vi "Harry_kane_CDR.vi"() -> ()   [LabVIEW 2013]
uses:
  <vilib>/vision/Image Controls.llb/IMAQ Image.ctl
  <vilib>/vision/driver/NI_Vision_Acquisition_Software.lvlib
panel:
  in  "Boolean":bool
  in  "stop":bool
  in  "Player area overlay":T1
  out "Puck and player location":T1(plugin-control)
  out "Player Array From Reference":dbl[][](array[numeric])
  out "Puck Array From Reference":dbl[][](array[numeric])
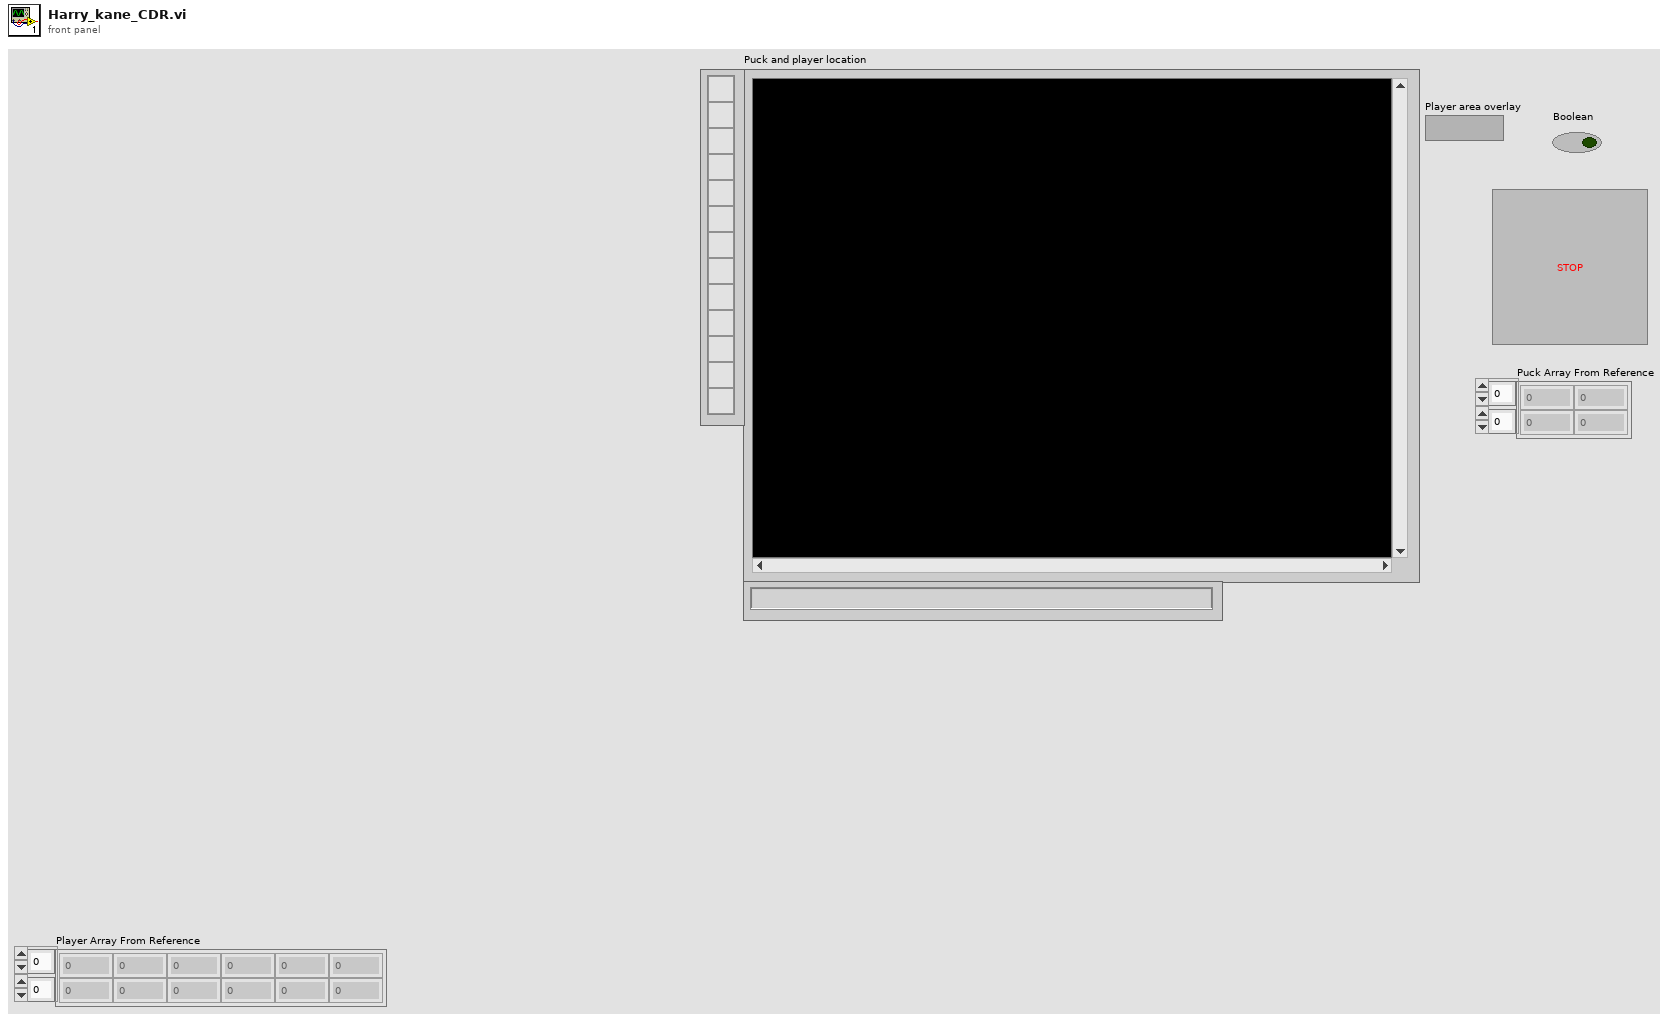
[diagram p1: front panel]
types:
  T1 = typedef "IMAQ Image.ctl" = refnum<image>
  T2 = typedef "Image Type" = u32
  T3 = typedef "IMAQdx.ctl" = refnum<k21>
  T4 = cluster{"Point1 (Pixels)":cluster{"X":sgl, "Y":sgl}, "Point2 (Pixels)":cluster{"X":sgl, "Y":sgl}, "Point1 (Real-World)":cluster{"X":sgl, "Y":sgl}, "Point2 (Real-World)":cluster{"X":sgl, "Y":sgl}, "Angle (Pixel)":dbl, "Angle (Real-World)":dbl, "Score":dbl, "Straightness":dbl, "Average SNR (db)":dbl, "Calibration Valid":bool}
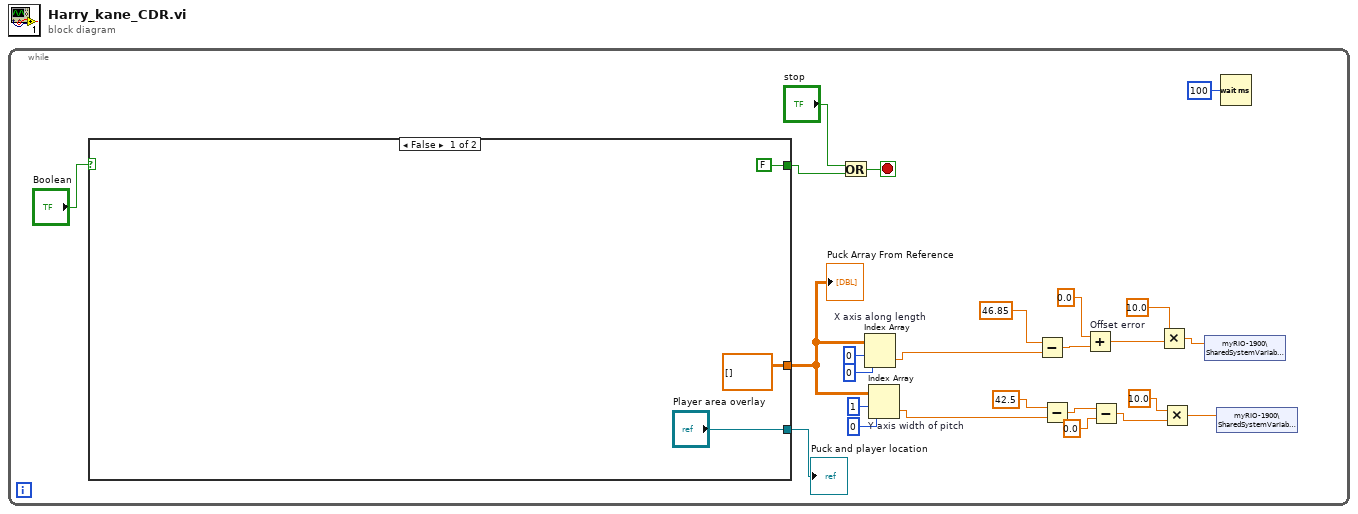
[diagram p0: block diagram]
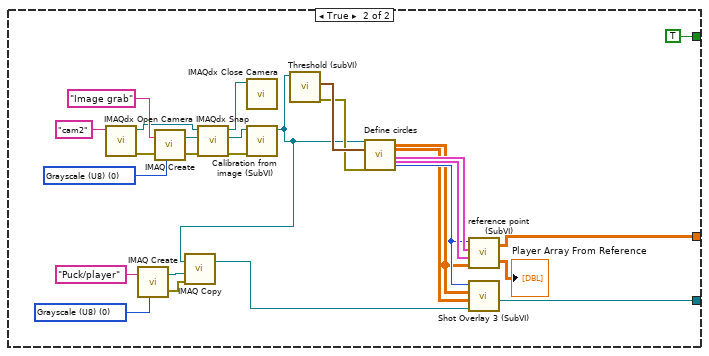
[diagram p2: hidden frame]
diagram:
  n1 = while {
    stop <- w15 stop-if-true
    n2 = case shown="False" "Boolean" {
      tunnel: ["Player area overlay" w37] -> w25
      tunnel: [dbl[][] [] ("Puck X, Y co-ordinates") w36] -> w22
      tunnel: [FALSE ("x") TRUE ("x")] -> w16
      frame False {
      }
      frame True {
        w32 = T2 0 items=["Grayscale (U8)", "Grayscale (I16)", "Grayscale (SGL)", "Complex (CSG)", "RGB (U32)", "HSL (U32)", "RGB (U64)", "Grayscale (U16)"] ("Image Type")
        w54 = T2 0 items=["Grayscale (U8)", "Grayscale (I16)", "Grayscale (SGL)", "Complex (CSG)", "RGB (U32)", "HSL (U32)", "RGB (U64)", "Grayscale (U16)"] ("Image Type")
        n3 = call <vilib>:"IMAQdx Open Camera.vi"("Session In"="cam2" ("Interface Name")) -> ("error out"=w48:errorcluster, "Session Out"=w49:T3)  [unwired: 9 in]
        n4 = call "IMAQ Create"("Image Name"="Puck/player", "Image Type"=w32) -> ("New Image"=w34:T1, "error out"=w33:errorcluster)  [unwired: 3 in]
        n5 = call "IMAQ Create"("Image Name"="Image grab", "Image Type"=w54, "error in (no error)"=w48) -> ("New Image"=w53:T1, "error out"=w52:errorcluster)  [unwired: 2 in]
        n6 = call <vilib>:"IMAQdx Snap.vi"("error in"=w52, "Image In"=w53, "Session In"=w49) -> ("error out"=w46:errorcluster, "Image Out"=w47:T1, "Session Out"=w51:T3)  [unwired: 6 in]
        n7 = call <vilib>:"IMAQdx Close Camera.vi"("Session In"=w51) -> ()  [unwired: 10 in, 1 out]
        n8 = call "Calibration from image (SubVI).vi"("error in (no error)"=w46, "Refnum in"=w47) -> ("Refnum out"=w30:T1)  [unwired: 8 in, 1 out]
        n9 = call "IMAQ Copy"("error in (no error)"=w33, "Image Dst"=w34, "Image Src"=w30) -> ("Image Dst Out"=w29:T1)  [unwired: 3 in, 1 out]
        n10 = call "Threshold (subVI).vi"("Image  in"=w30) -> ("error out"=w42:errorcluster, "Cluster"=w45:cluster{sgl, "element":sgl})  [unwired: 8 in, 1 out]
        n11 = call "Define circles"("Image In"=w30, "Range (Threshold 1)"=w45, "error in"=w42) -> ("Particle Measurements (Real-World) (Particle Analysis 1)"=w39:dbl[][], "Particle Measurements (Pixels) (Particle Analysis 1)"=w38:dbl[][], "Straight Edge (Find Straight Edge 1)"=w44:T4, "Straight Edge (Find Straight Edge 2)"=w43:T4, "Nb Circles (Circle Detection 1)"=w40:i32)  [unwired: 17 in, 3 out]
        n12 = call "reference point (SubVI).vi"("Nb Circles (Circle Detection 1)"=w40, "Straight Edge (Find Straight Edge 1)"=w44, "Straight Edge (Find Straight Edge 2)"=w43, "Particle Measurements (Real-World) (Particle Analysis 1)"=w39) -> ("Puck X, Y co-ordinates"=w36:dbl[][], "Player X, Y co-ordinates"=→"Player Array From Reference":dbl[][])  [unwired: 1 in]
        n13 = call "Shot Overlay 3 (SubVI).vi"("Image Out"=w29, "Particle Measurements (Pixels) (Particle Analysis 1)"=w38, "Particle Measurements (Real-World) (Particle Analysis 1)"=w39, "Nb Circles (Circle Detection 1)"=w40) -> ("Player area overlay"=w37:T1)  [unwired: 3 in, 2 out]
      }
    }
    "Puck and player location" <- w25
    "Puck Array From Reference" <- w22
    n14 = Or(x="stop", y=w16) -> (x .or. y?=w15:bool)
    n15 = Index Array "X axis along length"(array=w22, index (row)=0, index (col)=0 ("disabled index (col)")) -> (element=w19:dbl)
    n16 = Index Array "Y axis width of pitch"(array=w22, index (row)=1, index (col)=0 ("disabled index (col)")) -> (element=w8:dbl)
    n17 = Subtract(x=46.85, y=w19) -> (x-y=w14:dbl)
    n18 = Subtract(x=42.5, y=w8) -> (x-y=w9:dbl)
    n19 = Add "Offset error"(x=0.0, y=w14) -> (x+y=w6:dbl)
    n20 = Subtract(x=w9, y=0.0) -> (x-y=w3:dbl)
    n21 = Multiply(x=10.0, y=w6) -> (x*y=w5:dbl)
    n22 = Multiply(x=10.0, y=w3) -> (x*y=w2:dbl)
    n23 = shared-variable "myRIO-1900\\SharedSystemVariables.lvlib\\Puck Y"(w5) -> ()  [unwired: 1 in, 1 out]
    n24 = shared-variable "myRIO-1900\\SharedSystemVariables.lvlib\\Puck X"(w2) -> ()  [unwired: 1 in, 1 out]
    n25 = Wait (ms)(milliseconds to wait=u32 100) -> ()  [unwired: 1 out]
  }
